vi "DAQmxStatus-Com-Exec.vi"(8 "error in (no error)":errorcluster, 11 "DAQmxTaksContainer_General in":refnum<class "DAQmxTaksContainer_General.lvclass">) -> (0 "error out":errorcluster, 3 "DAQmxTaksContainer_General out":refnum<class "DAQmxTaksContainer_General.lvclass">)   [LabVIEW 2015, in "DAQmxTaksContainer_General.lvclass"]
uses:
  DAQmxTaksContainer_General.lvclass
  dependecies/ControlsVIs/Clusters-def/DAQmx-Reply-Connect-client.ctl
  dependecies/ControlsVIs/Clusters-def/SERVER-Commands.ctl
  dependecies/ControlsVIs/Clusters-def/Message types.ctl
  DAQmxTask.lvclass
  Control/Control-Server/Control-Server.lvclass
  Message/Message.lvclass
  GeneralFunctionality/GeneralFunctionality.lvclass
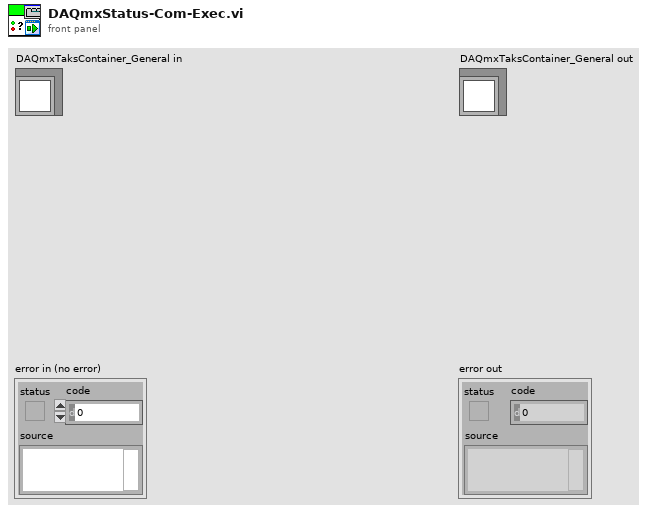
[diagram p1: front panel]
types:
  T1 = typedef "Message types.ctl" = string
  T2 = typedef "Control-Server.lvclass/SERVER-Commands.ctl" = string
  T3 = typedef "DAQmxTaksContainer_General.lvclass/DAQmx-Reply-Connect-client.ctl" = cluster{"on/off":bool, "RelayKeyHeater/off":bool, "LaserShutter":bool, "AcceleratorShutter":bool, "Power":bool, "Faraday Cup Status":bool, "error":errorcluster}
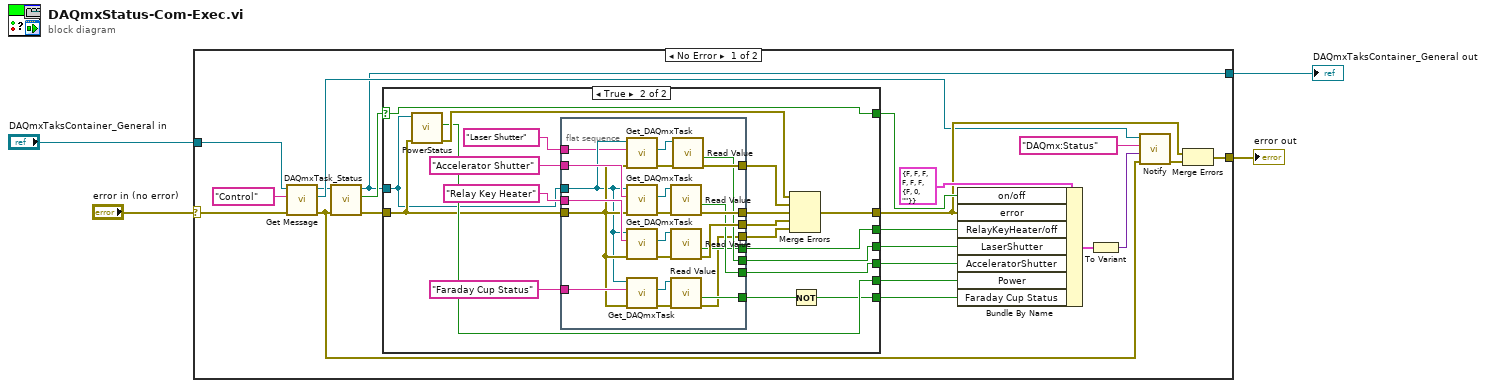
[diagram p0: block diagram]
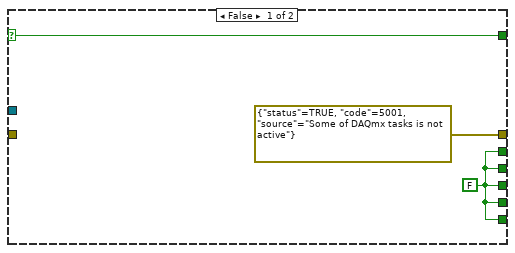
[diagram p2: hidden frame]
diagram:
  n1 = case shown="No Error" "error in (no error)" {
    selector: "error in (no error)" -> [w17 w72]
    tunnel: [w12 w72] -> w4
    tunnel: [w5 w71] -> w3
    tunnel: "DAQmxTaksContainer_General in" -> [w9 w71]
    frame No Error {
      n2 = call "Get Message.vi"("error in (no error)"=w17, "Message type"=T1 "Control", "GeneralFunctionality en entrée"=w9) -> ("error out"=w7:errorcluster, "Message.lvclass"=w16:refnum<class "Message.lvclass">, "GeneralFunctionality en sortie"=w8:refnum<class "DAQmxTaksContainer_General.lvclass">)  [unwired: 6 in]
      n3 = call-dynamic "DAQmxTask_Status.vi"("error in (no error)"=w7, "DAQmxTaskContainer_General en entrée"=w8) -> ("error out"=w21:errorcluster, "All active"=w6:bool, "DAQmxTaskContainer_General en sortie"=w5:refnum<class "DAQmxTaksContainer_General.lvclass">)  [unwired: 6 in, 1 out]
      n4 = case shown="True" w6 {
        selector: w6 -> [w28 w36]
        tunnel: [errorcluster {"status"=TRUE, "code"=5001, "source"="Some of DAQmx tasks is not active"} ("error IO") w42] -> w19
        tunnel: [w27 w37] -> w22
        tunnel: [w27 w41] -> w23
        tunnel: [w27 w40] -> w24
        tunnel: [w27 w39] -> w25
        tunnel: w21 -> [_ w34]
        tunnel: w5 -> [_ w31]
        tunnel: [w28 w36] -> w20
        tunnel: [w27 w30] -> w10
        frame False {
          w27 = FALSE ("Data")
        }
        frame True {
          n5 = call "PowerStatus.vi"("error in (no error)"=w34, "DAQmxTaskContainer_General in"=w31) -> ("error out"=w38:errorcluster, "On/Off"=w37:bool)  [unwired: 7 in, 1 out]
          n6 = flat-sequence {
            tunnel: [w70] -> w48
            tunnel: [w69] -> w47
            tunnel: [w68] -> w46
            tunnel: "Relay Key Heater" ("Task name") -> [w61]
            tunnel: "Accelerator Shutter" ("Task name") -> [w60]
            tunnel: "Laser Shutter" ("Task name") -> [w49]
            tunnel: [w59] -> w41
            tunnel: [w58] -> w40
            tunnel: [w57] -> w39
            tunnel: "Faraday Cup Status" ("Task name") -> [w55]
            tunnel: w34 -> [w54]
            tunnel: [w53] -> w33
            tunnel: [w51] -> w32
            tunnel: w31 -> [w50]
            frame #0 {
              n7 = call "Get_DAQmxTask.vi"("error in (no error)"=w54, "Task name"=w49, "DAQmxTaksContainer_General in"=w50) -> ("error out"=w62:errorcluster, "DAQmx Task"=w63:refnum<class "DAQmxTask.lvclass">)  [unwired: 6 in, 1 out]
              n8 = call "Get_DAQmxTask.vi"("error in (no error)"=w54, "Task name"=w60, "DAQmxTaksContainer_General in"=w50) -> ("error out"=w64:errorcluster, "DAQmx Task"=w65:refnum<class "DAQmxTask.lvclass">)  [unwired: 6 in, 1 out]
              n9 = call "Get_DAQmxTask.vi"("error in (no error)"=w54, "Task name"=w61, "DAQmxTaksContainer_General in"=w50) -> ("error out"=w66:errorcluster, "DAQmx Task"=w67:refnum<class "DAQmxTask.lvclass">)  [unwired: 6 in, 1 out]
              n10 = call "Get_DAQmxTask.vi"("error in (no error)"=w54, "Task name"=w55, "DAQmxTaksContainer_General in"=w50) -> ("error out"=w52:errorcluster, "DAQmx Task"=w56:refnum<class "DAQmxTask.lvclass">)  [unwired: 6 in, 1 out]
              n11 = call-dynamic "Read Value.vi"("error in (no error)"=w64, "DAQmxTask en entrée"=w65) -> ("error out"=w69:errorcluster, "Data"=w58:bool)  [unwired: 6 in, 2 out]
              n12 = call-dynamic "Read Value.vi"("error in (no error)"=w66, "DAQmxTask en entrée"=w67) -> ("error out"=w70:errorcluster, "Data"=w57:bool)  [unwired: 6 in, 2 out]
              n13 = call-dynamic "Read Value.vi"("error in (no error)"=w52, "DAQmxTask en entrée"=w56) -> ("error out"=w51:errorcluster, "Data"=w53:bool)  [unwired: 6 in, 2 out]
              n14 = call-dynamic "Read Value.vi"("error in (no error)"=w62, "DAQmxTask en entrée"=w63) -> ("error out"=w68:errorcluster, "Data"=w59:bool)  [unwired: 6 in, 2 out]
            }
          }
          n15 = Merge Errors(w38, w46, w47, w48, w32) -> (w42:errorcluster)
          n16 = Not(x=w33) -> (.not. x?=w30:bool)
        }
      }
      n17 = Bundle By Name(cluster=T3 {"on/off"=FALSE, "RelayKeyHeater/off"=FALSE, "LaserShutter"=FALSE, "AcceleratorShutter"=FALSE, "Power"=FALSE, "Faraday Cup Status"=FALSE, "error"={"status"=FALSE, "code"=0, "source"=""}} ("output cluster"), "on/off"=w20, "error"=w19, "RelayKeyHeater/off"=w25, "LaserShutter"=w23, "AcceleratorShutter"=w24, "Power"=w22, "Faraday Cup Status"=w10) -> (w18:T3)
      n18 = To Variant(anything=w18) -> (Variant=w15:variant)
      n19 = call "Notify.vi"("error in (no error)"=w7, "Data"=w15, "command"=T2 "DAQmx:Status" ("Commands"), "Message en entrée"=w16) -> ("error out"=w13:errorcluster)  [unwired: 6 in, 1 out]
      n20 = Merge Errors(w19, w13) -> (w12:errorcluster)
    }
    frame Error {
    }
  }
  "error out" <- w4
  "DAQmxTaksContainer_General out" <- w3
